vi "Concatenate Output.vi"() -> ()   [LabVIEW 2015]
uses:
  <vilib>/measure/NI_MABase.lvlib
panel:
  out "Waveform Graph":dbl[](graph)
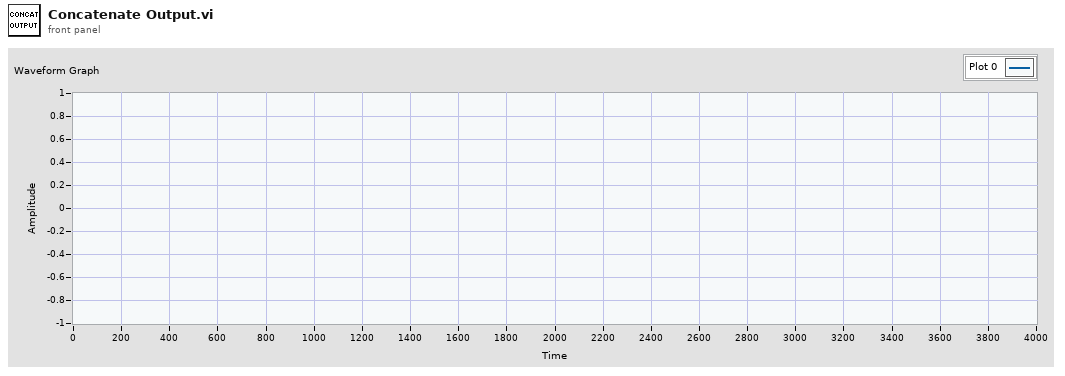
[diagram p1: front panel]
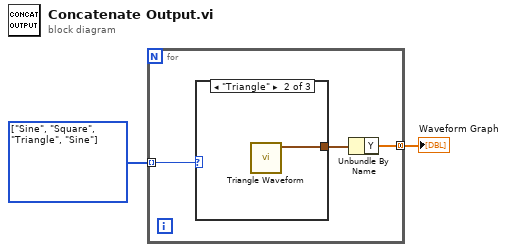
[diagram p0: block diagram]
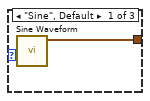
[diagram p2: hidden frame]
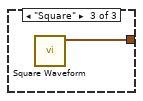
[diagram p3: hidden frame]
diagram:
  w2 = enum16{"Sine", "Triangle", "Square"}[] [enum."Sine", enum."Square", enum."Triangle", enum."Sine"] items=["Sine", "Triangle", "Square"]
  n1 = for {
    tunnel: w2 -> [w5] mode=indexing
    tunnel: [w3] -> w1 mode=concatenating
    n2 = case shown="\"Triangle\"" w5 {
      tunnel: [w6 w7 w8] -> w4
      frame "Sine", Default {
        n3 = call <vilib>:"Sine Waveform.vi"() -> ("signal out"=w6:waveform(dbl))  [unwired: 10 in, 1 out]
      }
      frame "Triangle" {
        n4 = call <vilib>:"Triangle Waveform.vi"() -> ("signal out"=w7:waveform(dbl))  [unwired: 10 in, 1 out]
      }
      frame "Square" {
        n5 = call <vilib>:"Square Waveform.vi"() -> ("signal out"=w8:waveform(dbl))  [unwired: 10 in, 1 out]
      }
    }
    n6 = Unbundle By Name(w4) -> ("Y"=w3:dbl[])
  }
  "Waveform Graph" <- w1
